vi "Load Sample Catagory.vi"(8 "error in (no error)":errorcluster, 10 "Item List":T1, 11 "TreeControl in":refnum<vi>) -> (0 "error out":errorcluster)   [LabVIEW 2021]
uses:
  Control/Item List.ctl
  Control/Item Info.ctl
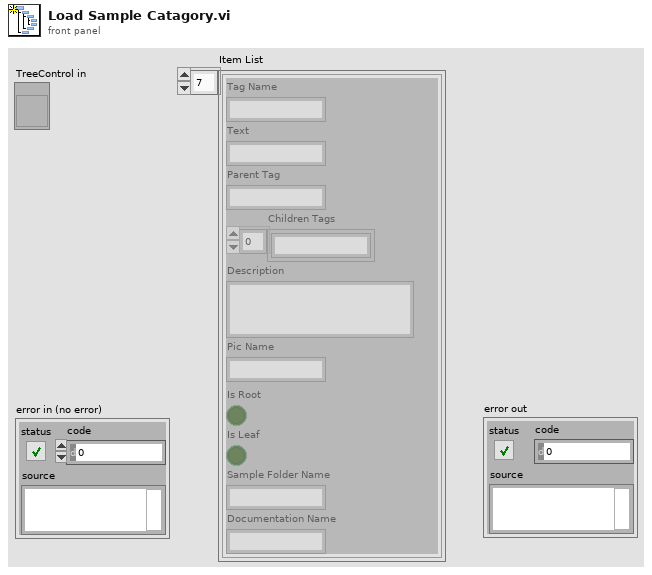
[diagram p1: front panel]
types:
  T1 = typedef "Item List.ctl" = T2[]
  T2 = typedef "Item Info.ctl" = cluster{"Tag Name":string, "Text":string, "Parent Tag":string, "Children Tags":string[], "Description":string, "Pic Name":string, "Is Root":bool, "Is Leaf":bool, "Sample Folder Name":string, "Documentation Name":string}
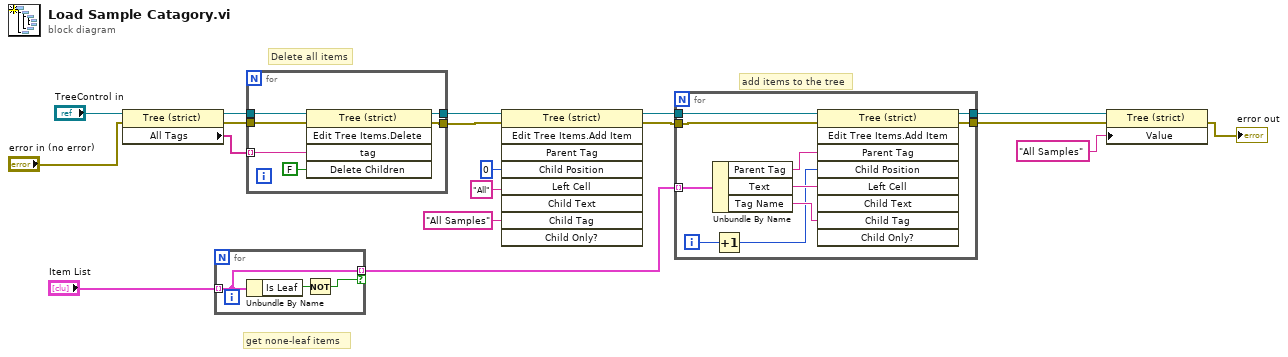
[diagram p0: block diagram]
diagram:
  # "add items to the tree"
  # "get none-leaf items"
  # "Delete all items"
  n1 = property class="Tree (strict)"(reference="TreeControl in", error in="error in (no error)") -> (reference out=w17:refnum<vi>, error out=w8:errorcluster, "All Tags"=w16:string[])
  n2 = for {
    tunnel: "Item List" -> [w21] mode=indexing
    tunnel: [w21] -> w14 mode=indexing if=w19
    n3 = Unbundle By Name(w21) -> ("Is Leaf"=w20:bool)
    n4 = Not(x=w20) -> (.not. x?=w19:bool)
  }
  n5 = for {
    tunnel: w16 -> [w27] mode=indexing
    tunnel: w17 -> [w25]
    tunnel: [w24] -> w13
    tunnel: w8 -> [w23]
    tunnel: [w22] -> w7
    n6 = invoke on="Invoke Node" class="Tree (strict)" method="Edit Tree Items.Delete"(reference=w25, error in=w23, "tag"=w27, "Delete Children"=FALSE ("Delete Children?")) -> (reference out=w24:refnum<vi>, error out=w22:errorcluster)  [unwired: 1 in, 3 out]
  }
  n7 = invoke class="Tree (strict)" method="Edit Tree Items.Add Item"(reference=w13, error in=w7, "Child Position"=0, "Left Cell"="All" ("Left Cell String"), "Child Tag"="All Samples") -> (reference out=w12:refnum<vi>, error out=w6:errorcluster)  [unwired: 4 in, 7 out]
  n8 = for {
    tunnel: w14 -> [w37] mode=indexing
    tunnel: w12 -> [w33]
    tunnel: w6 -> [w30]
    tunnel: [w29] -> w3
    tunnel: [w28] -> w4
    i -> [w32]
    n9 = Unbundle By Name(w37) -> ("Parent Tag"=w35:string, "Text"=w36:string, "Tag Name"=w34:string)
    n10 = Increment(x=w32) -> (x+1=w31:i32)
    n11 = invoke on="Invoke Node" class="Tree (strict)" method="Edit Tree Items.Add Item"(reference=w33, error in=w30, "Parent Tag"=w35, "Child Position"=w31, "Left Cell"=w36, "Child Tag"=w34) -> (reference out=w28:refnum<vi>, error out=w29:errorcluster)  [unwired: 3 in, 7 out]
  }
  n12 = property class="Tree (strict)"(reference=w4, error in=w3, "Value"="All Samples" ("Active Cell:String")) -> (error out=→"error out":errorcluster)  [unwired: 1 out]
